vi "Fetch FFT Measurement Peak Search Result.vi"(8 "error in (no error)":errorcluster, 9 "Result Type (Current)":i32(ring) items=["Current", "Average"], 10 "Instance (1)":i32=1, 11 "VISA resource name":refnum<visa-resource-name>) -> (0 "error out":errorcluster, 1 "Power":dbl[](array[numeric]) format="%^.3e", 2 "Reliability":i32, 3 "VISA resource name out":refnum<visa-resource-name>, 4 "Frequency":dbl[](array[numeric]) format="%#.9p")   [LabVIEW 2015, in "Rohde&Schwarz CMXP GPRF.lvlib"]
doc: "Returns the results of the peak search.\n\nAttributes:\nRSCMXPGPRF_ATTR_FETCH_FFT_MEASUREMENT_PEAK_SEARCH_RESULT_CURRENT\nRSCMXPGPRF_ATTR_FETCH_FFT_MEASUREMENT_PEAK_SEARCH_RESULT_AVERAGE\n\nRemote-control commands:\nFETCh:GPRF:MEAS<i>:FFTSanalyzer:PEAKs:CURRent?\nFETCh:GPRF:MEAS<i>:FFTSanalyzer:PEAKs:AVERage?"
uses:
  <instrlib>/Rohde&Schwarz CMXP GPRF/Rohde&Schwarz CMXP GPRF.lvlib
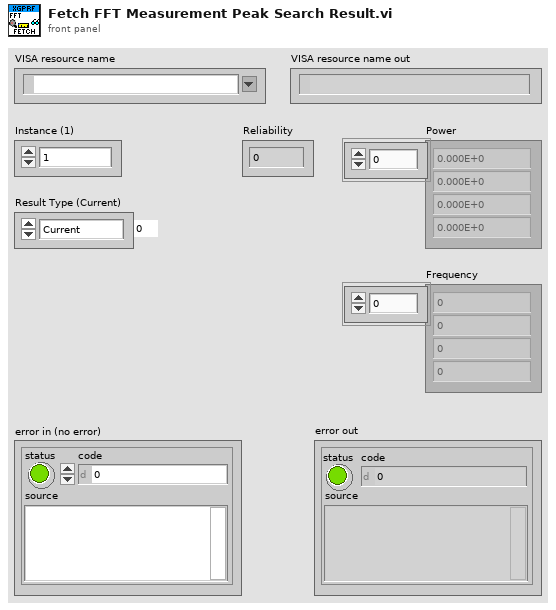
[diagram p1: front panel]
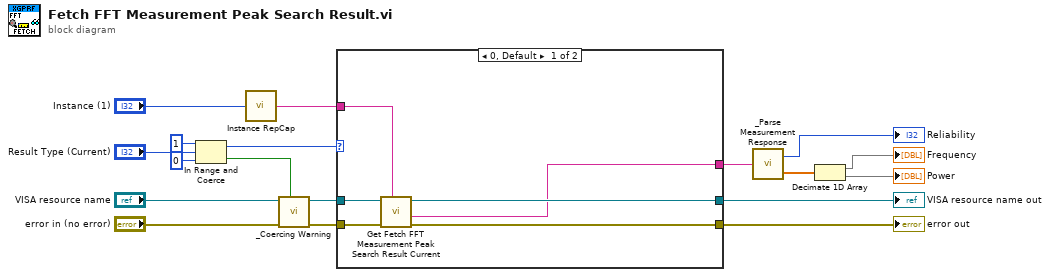
[diagram p0: block diagram]
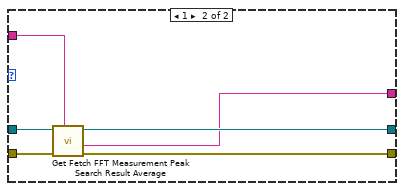
[diagram p2: hidden frame]
diagram:
  n1 = In Range and Coerce(upper limit=1, x="Result Type (Current)", lower limit=0) -> (coerced(x)=w15:i32, In Range?=w5:bool)
  n2 = call <instrlib>:"Instance RepCap.vi"("instance  in"="Instance (1)") -> ("instance out"=w16:string)
  n3 = call <instrlib>:"_Coercing Warning.vi"("In Range?"=w5, "error in (no error)"="error in (no error)", "VISA resource name"="VISA resource name") -> ("error out"=w14:errorcluster, "VISA resource name out"=w13:refnum<visa-resource-name>)  [unwired: 7 in]
  n4 = case shown="0, Default" w15 {
    tunnel: w16 -> [w20 w26]
    tunnel: w14 -> [w24 w30]
    tunnel: w13 -> [w23 w29]
    tunnel: [w22 w28] -> w9
    tunnel: [w21 w27] -> w8
    tunnel: [w19 w25] -> w1
    frame 0, Default {
      n5 = call "Get Fetch FFT Measurement Peak Search Result Current"("Repeated Capabilities"=w20, "error in (no error)"=w24, "instrument handle"=w23) -> ("error out"=w22:errorcluster, "Fetch FFT Measurement Peak Search Result Current"=w19:string, "instrument handle out"=w21:refnum<visa-resource-name>)  [unwired: 6 in]
    }
    frame 1 {
      n6 = call "Get Fetch FFT Measurement Peak Search Result Average"("Repeated Capabilities"=w26, "error in (no error)"=w30, "instrument handle"=w29) -> ("error out"=w28:errorcluster, "Fetch FFT Measurement Peak Search Result Average"=w25:string, "instrument handle out"=w27:refnum<visa-resource-name>)  [unwired: 6 in]
    }
  }
  "error out" <- w9
  "VISA resource name out" <- w8
  n7 = call <instrlib>:"_Parse Measurement Response.vi"("String In"=w1) -> ("Reliability"=→"Reliability":i32, "Data"=w3:dbl[])
  n8 = Decimate 1D Array(w3) -> (→"Frequency":dbl[], →"Power":dbl[])
